vi "临时.vi"() -> ()   [LabVIEW 2011]
panel:
  in  "基路径":path
  in  "DBSet":T1={"Server"="172.20.23.107", "DB"="MESDATACenter", "PSW"="data'songyy", "User"="sa"}
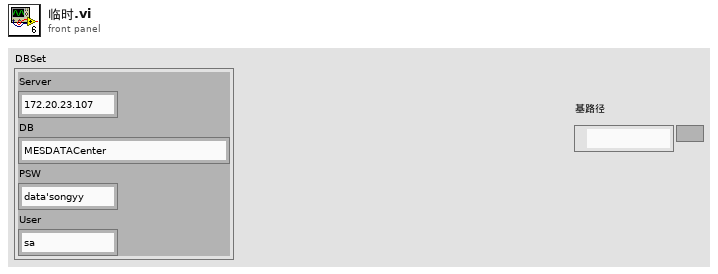
[diagram p1: front panel]
types:
  T1 = cluster{"Server":string, "DB":string, "PSW":string, "User":string}
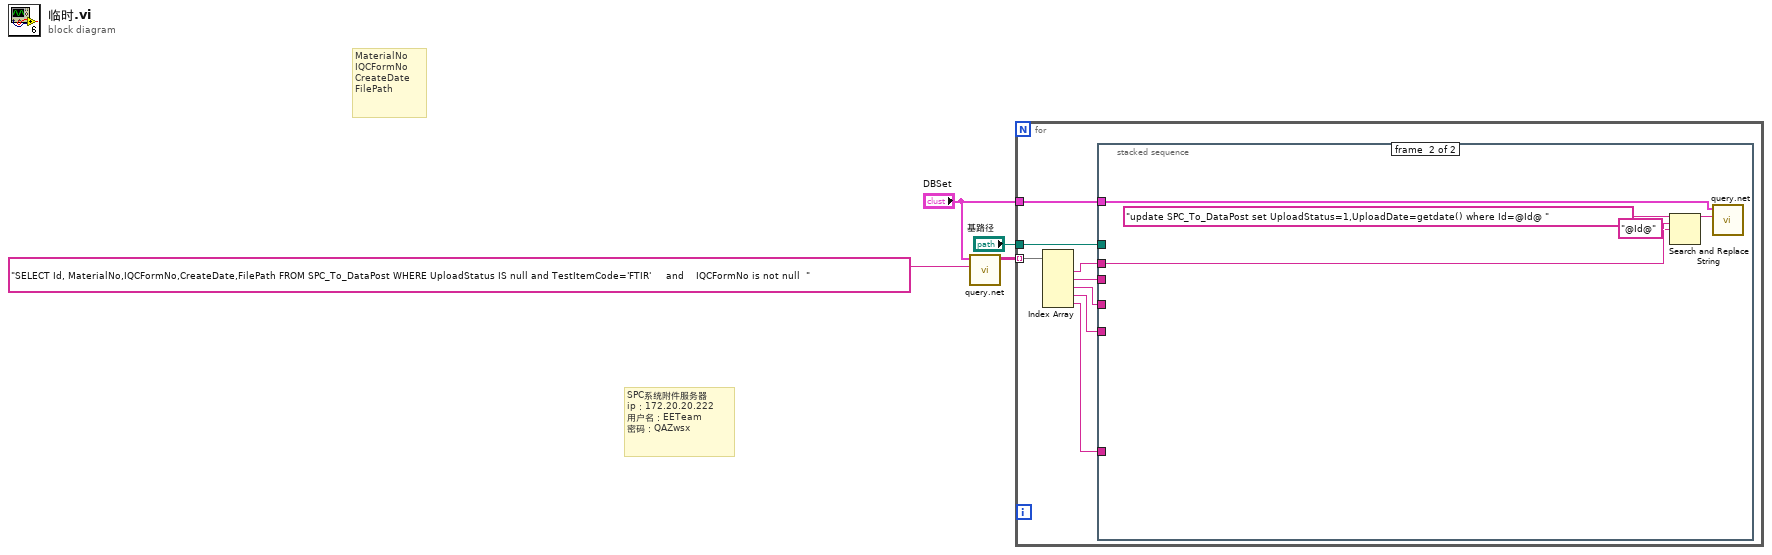
[diagram p0: block diagram]
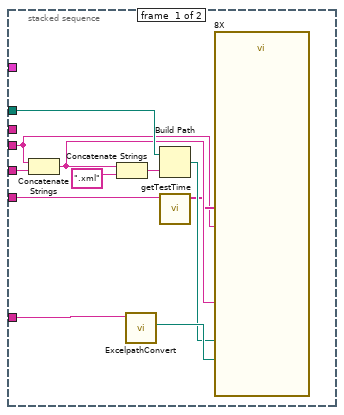
[diagram p2: hidden frame]
diagram:
  # "SPC系统附件服务器\nip：172.20.20.222\n用户名：EETeam\n密码：QAZwsx"
  # "MaterialNo\nIQCFormNo\nCreateDate\nFilePath"
  n1 = call "query.net.vi"("Sql"="SELECT Id, MaterialNo,IQCFormNo,CreateDate,FilePath FROM SPC_To_DataPost WHERE UploadStatus IS null and TestItemCode='FTIR'     and    IQCFormNo is not null  ", "DBSet"="DBSet") -> ("result"=w3:string[][])  [unwired: 8 in, 1 out]
  n2 = for {
    tunnel: w3 -> [w12] mode=indexing
    tunnel: "基路径" -> [w10]
    tunnel: "DBSet" -> [w5]
    n3 = Index Array(array=w12) -> (element #1=w6:string, element #2=w7:string, element #3=w9:string, element #4=w8:string, element #5=w11:string)  [unwired: 5 in]
    n4 = stacked-sequence {
      tunnel: w11 -> [w23 _]
      tunnel: w10 -> [w21 _]
      tunnel: w9 -> [w20 _]
      tunnel: w8 -> [w15 _]
      tunnel: w7 -> [w13 _]
      tunnel: w6 -> [_ w24]
      tunnel: w5 -> [_ w28]
      frame #0 {
        n5 = Concatenate Strings(w13, w20) -> (w19:string)
        n6 = Concatenate Strings(w19, ".xml" ("字符串")) -> (w17:string)
        n7 = call "ExcelpathConvert.vi"("输入字符串"=w23) -> ("路径"=w22:path)  [unwired: 9 in, 1 out]
        n8 = Build Path(base path=w21, name or relative path=w17) -> (appended path=w16:path)
        n9 = call "getTestTime.vi"("startTime"=w15) -> ("timeArray"=w14:string[])  [unwired: 9 in, 1 out]
        n10 = call "8X.vi"("input_str_CustomerPN"=w13, "SN"=w19, "文件路径"=w22, "input_array_time"=w14, "xml path"=w16) -> ()  [unwired: 14 in, 1 out]
      }
      frame #1 {
        n11 = Search and Replace String(input string="update SPC_To_DataPost set UploadStatus=1,UploadDate=getdate() where Id=@Id@ " ("Sql"), search string="@Id@" ("搜索字符串"), replace string=w24) -> (result string=w26:string)  [unwired: 5 in, 3 out]
        n12 = call "query.net.vi"("Sql"=w26, "DBSet"=w28) -> ()  [unwired: 8 in, 2 out]
      }
    }
  }
